vi "Configure Offset and Limits (Demodulation - AM).vi"(0 "VISA resource name":refnum<visa-resource-name>, 1 "AM Depth Upper (100 percentage)":dbl=100.0, 3 "Carrier Frequency Offset Upper (1E+6 Hz)":dbl=1000000.0, 5 "Enable Limit (F: Disable)":bool, 9 "Carrier Power Upper (10 dBm)":dbl=10.0, 11 "error in (no error)":errorcluster, 12 "AM Depth Lower (0.1 percentage)":dbl=0.1) -> (4 "VISA resource name out":refnum<visa-resource-name>, 15 "error out":errorcluster)   [LabVIEW 2022 SP3, in "Agilent N934X Series.lvlib"]
doc: "Configures the general setting for AM demodulation offset and limits of Demodulation Option.\n\nNote:\nThis VI is only applicable for N9321C, N9322C, N9323C, N9324C models."
uses:
  <instrlib>/Agilent N934X Series/Agilent N934X Series.lvlib
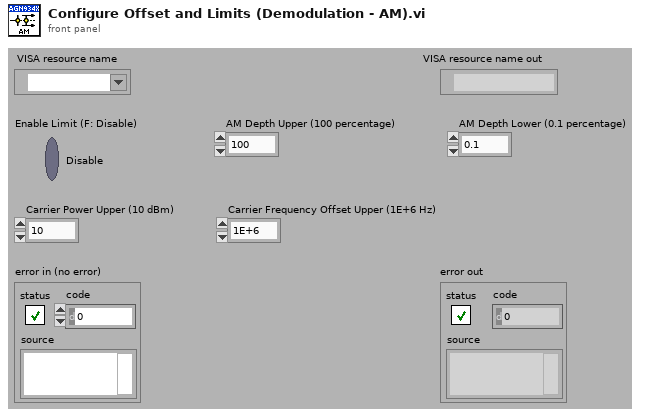
[diagram p1: front panel]
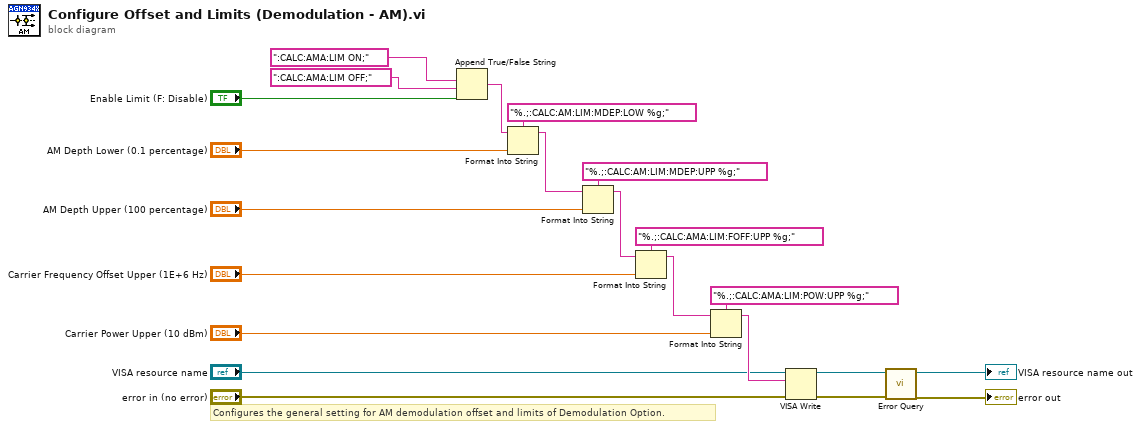
[diagram p0: block diagram]
diagram:
  # "Configures the general setting for AM demodulation offset and limits of Demodulation Option."
  n1 = Append True/False String(1:"Enable Limit (F: Disable)", 2:":CALC:AMA:LIM OFF;", 3:":CALC:AMA:LIM ON;") -> (0:w1:string)  [unwired: 1 in]
  n2 = Format Into String(format string="%.;:CALC:AM:LIM:MDEP:LOW %g;", initial string=w1, "AM Depth Lower (0.1 percentage)") -> (resulting string=w20:string)  [unwired: 1 in, 1 out]
  n3 = Format Into String(format string="%.;:CALC:AM:LIM:MDEP:UPP %g;", initial string=w20, "AM Depth Upper (100 percentage)") -> (resulting string=w2:string)  [unwired: 1 in, 1 out]
  n4 = Format Into String(format string="%.;:CALC:AMA:LIM:FOFF:UPP %g;", initial string=w2, "Carrier Frequency Offset Upper (1E+6 Hz)") -> (resulting string=w12:string)  [unwired: 1 in, 1 out]
  n5 = Format Into String(format string="%.;:CALC:AMA:LIM:POW:UPP %g;", initial string=w12, "Carrier Power Upper (10 dBm)") -> (resulting string=w9:string)  [unwired: 1 in, 1 out]
  n6 = VISA Write(VISA resource name="VISA resource name", write buffer=w9, error in (no error)="error in (no error)") -> (VISA resource name out=w6:refnum<visa-resource-name>, error out=w5:errorcluster)  [unwired: 1 out]
  n7 = call <instrlib>:"Error Query.vi"("error in (no error)"=w5, "VISA resource name"=w6) -> ("error out"=→"error out":errorcluster, "VISA resource name out"=→"VISA resource name out":refnum<visa-resource-name>)  [unwired: 6 in, 2 out]
